vi "waitNotifierStopServer.vi"(8 "error in (no error)":errorcluster, 11 "TcpServerBase in":refnum<class "TcpServerBase.lvclass">) -> (0 "error out":errorcluster, 2 "stopServer":bool, 3 "TcpServerBase out":refnum<class "TcpServerBase.lvclass">)   [LabVIEW 2018, in "TcpServerBase.lvclass"]
doc: "Wait for the notifierStopServer. This is a non-block call function.\n\nNOTE: put the VI in preallocated reentrant clone execution."
uses:
  TcpServerBase.lvclass
  TcpServerBase.lvclass/TcpServerBase.ctl
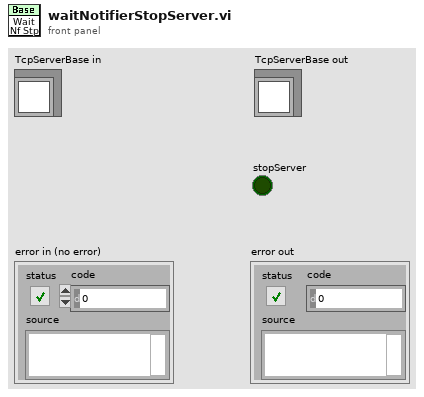
[diagram p1: front panel]
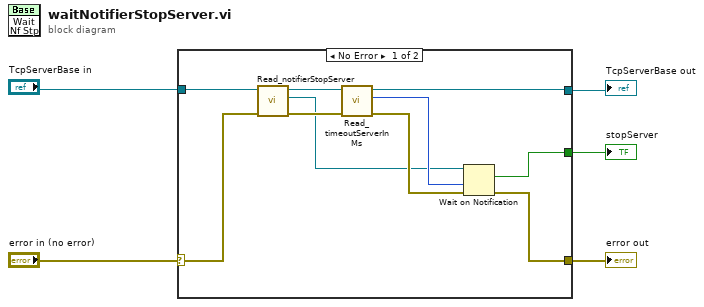
[diagram p0: block diagram]
diagram:
  n1 = case shown="No Error" "error in (no error)" {
    selector: "error in (no error)" -> [w15 w17]
    tunnel: "TcpServerBase in" -> [w8 w16]
    tunnel: [w11 w17] -> w4
    tunnel: [w14 w16] -> w1
    tunnel: [w10 _] -> w3
    frame No Error {
      n2 = call "Read_notifierStopServer.vi"("error in (no error)"=w15, "TcpServerBase in"=w8) -> ("error out"=w9:errorcluster, "notifierStopServer"=w6:refnum<notifier>, "TcpServerBase out"=w7:refnum<class "TcpServerBase.lvclass">)  [unwired: 7 in]
      n3 = call "Read_timeoutServerInMs.vi"("error in (no error)"=w9, "TcpServerBase in"=w7) -> ("error out"=w12:errorcluster, "timeoutServerInMs"=w13:i32, "TcpServerBase out"=w14:refnum<class "TcpServerBase.lvclass">)  [unwired: 7 in]
      n4 = Wait on Notification(notifier=w6, timeout in ms (-1)=w13, error in (no error)=w12) -> (notification=w10:bool, error out=w11:errorcluster)  [unwired: 1 in, 2 out]
    }
    frame Error {
    }
  }
  "error out" <- w4
  "stopServer" <- w3
  "TcpServerBase out" <- w1
